vi "UpdateData_Wrapper.vi"(6 "50mA Spectra":cluster{"Wavelength":dbl[], "EL Spectrum":dbl[]}, 7 "20mA Spectra":cluster{"Wavelength":dbl[], "EL Spectrum":dbl[]}, 8 "error in (no error)":errorcluster, 10 "Data In":T1 {"50mA Data"."Current,mA" format="%_6g"; "50mA Data"."WL" format="%_6g"; "50mA Data"."Voltage" format="%_6g"; "50mA Data"."Power" format="%_6g"; "20mA Data"."Reverse" format="%#_3g"; "20mA Data"."Current,mA" format="%_6g"; "20mA Data"."Knee Current" format="%#_3g"; "20mA Data"."WL" format="%_6g"; "20mA Data"."Voltage" format="%_6g"; "20mA Data"."Power" format="%_5g"}, 11 "EpiWrapper in":refnum<class "EpiWrapper.lvclass">) -> (0 "error out":errorcluster, 3 "EpiWrapper out":refnum<class "EpiWrapper.lvclass">)   [LabVIEW 2012, in "EpiWrapper.lvclass"]
uses:
  EpiWrapper.lvclass
  Controls/TestData.ctl
  EpiWrapper.lvclass/EpiWrapper.ctl
  LotData.lvclass
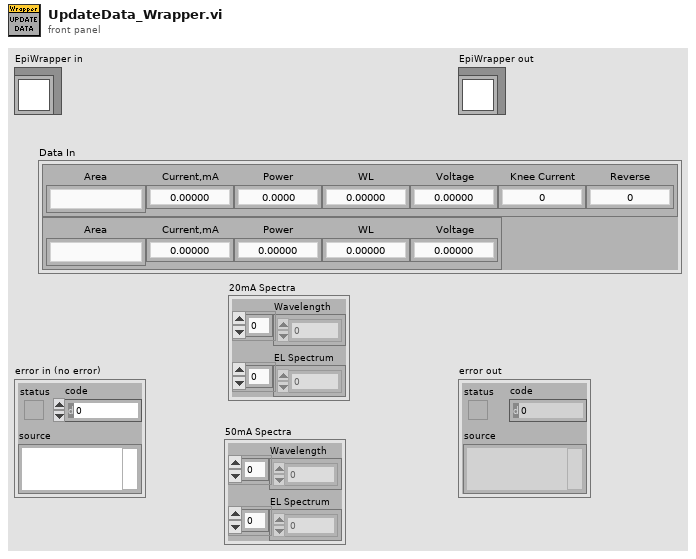
[diagram p1: front panel]
types:
  T1 = typedef "TestData.ctl" = cluster{"20mA Data":cluster{"Area":string, "Current,mA":dbl, "Power":dbl, "WL":dbl, "Voltage":dbl, "Knee Current":dbl, "Reverse":dbl}, "50mA Data":cluster{"Area":string, "Current,mA":dbl, "Power":dbl, "WL":dbl, "Voltage":dbl}}
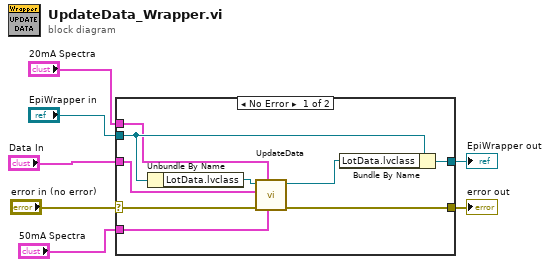
[diagram p0: block diagram]
diagram:
  n1 = case shown="No Error" "error in (no error)" {
    selector: "error in (no error)" -> [w13 w18]
    tunnel: [w8 w18] -> w6
    tunnel: [w10 w17] -> w4
    tunnel: "EpiWrapper in" -> [w15 w17]
    tunnel: "Data In" -> [w11 _]
    tunnel: "20mA Spectra" -> [w12 _]
    tunnel: "50mA Spectra" -> [w9 _]
    frame No Error {
      n2 = Unbundle By Name(w15) -> ("LotData.lvclass"=w16:refnum<class "LotData.lvclass">)
      n3 = call-dynamic "UpdateData.vi"("50mA Spectra"=w9, "20mA Spectra"=w12, "error in (no error)"=w13, "Data In"=w11, "LotData in"=w16) -> ("error out"=w8:errorcluster, "LotData out"=w14:refnum<class "LotData.lvclass">)  [unwired: 4 in, 1 out]
      n4 = Bundle By Name(cluster=w15, "LotData.lvclass"=w14) -> (w10:refnum<class "EpiWrapper.lvclass">)
    }
    frame Error {
    }
  }
  "error out" <- w6
  "EpiWrapper out" <- w4
